vi "led4.vi"() -> ()   [LabVIEW 2014]
panel:
  out "led4":bool
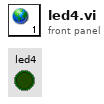
[diagram p1: front panel]
diagram:
